vi "scottSSObs.vi"(7 "Observer Variables":T1, 10 "u":dbl, 11 "y":dbl) -> (0 "xhat":dbl[](array[numeric]), 3 "-Kx":dbl)   [LabVIEW 2018, in "kevLib2010.lvlib"]
uses:
  kevLib2010.lvlib
  <vilib>/Analysis/baseanly.llb/Real Dot Product.vi
  <vilib>/Analysis/baseanly.llb/A x Vector.vi
  <vilib>/Analysis/NI_AALBase.lvlib
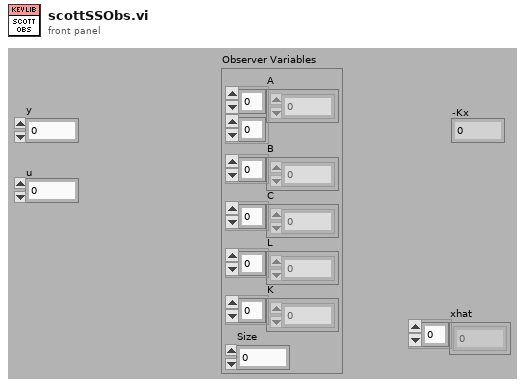
[diagram p1: front panel]
types:
  T1 = cluster{"A":dbl[][], "B":dbl[], "C":dbl[], "L":dbl[], "K":dbl[], "Size":dbl}
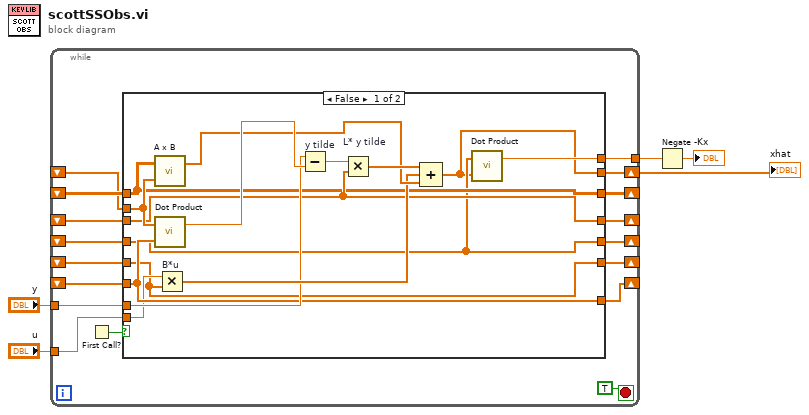
[diagram p0: block diagram]
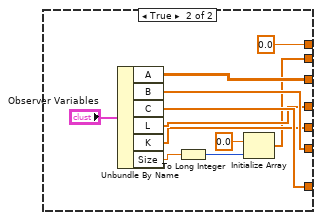
[diagram p2: hidden frame]
diagram:
  n1 = while {
    shift-right: [w20] -> _
    shift-left: _ -> [w15]
    shift-right: [w19] -> _
    shift-left: _ -> [w14]
    shift-right: [w18] -> _
    shift-left: _ -> [w13]
    shift-right: [w17] -> _
    shift-left: _ -> [w12]
    shift-right: [w16] -> _
    shift-left: _ -> [w11]
    shift-right: [w10] -> w1
    shift-left: _ -> [w9]
    tunnel: "y" -> [w8]
    tunnel: "u" -> [w7]
    tunnel: [w6] -> w3
    stop <- TRUE stop-if-true
    n2 = First Call?() -> (First Call?: T/F=w21:bool)
    n3 = case shown="False" w21 {
      tunnel: [w28 w47] -> w20
      tunnel: [w26 w46] -> w19
      tunnel: [w29 w45] -> w18
      tunnel: [w30 w44] -> w17
      tunnel: [w25 w43] -> w16
      tunnel: w15 -> [w28 _]
      tunnel: w14 -> [w26 _]
      tunnel: w13 -> [w29 _]
      tunnel: w12 -> [w30 _]
      tunnel: w11 -> [w25 _]
      tunnel: [w23 w39] -> w10
      tunnel: w9 -> [w31 _]
      tunnel: w8 -> [w32 _]
      tunnel: w7 -> [w27 _]
      tunnel: [w24 0.0 ("X * Y")] -> w6
      frame False {
        n4 = call-poly <vilib>:"A x B.vi"("Vector"=w31, "A"=w28) -> ("A x Vector"=w35:dbl[])  [unwired: 1 out]
        n5 = call-poly <vilib>:"Dot Product.vi"("Y Vector"=w29, "X Vector"=w31) -> ("X * Y"=w37:dbl)  [unwired: 1 out]
        n6 = Multiply "B*u"(x=w27, y=w26) -> (x*y=w34:dbl[])
        n7 = Subtract "y tilde"(x=w32, y=w37) -> (x-y=w33:dbl)
        n8 = Multiply "L* y tilde"(x=w33, y=w30) -> (x*y=w36:dbl[])
        n9 = Compound Arithmetic op=ADD(w36, w34, w35) -> (w23:dbl[])
        n10 = call-poly <vilib>:"Dot Product.vi"("Y Vector"=w23, "X Vector"=w25) -> ("X * Y"=w24:dbl)  [unwired: 1 out]
      }
      frame True {
        n11 = Unbundle By Name("Observer Variables") -> ("A"=w47:dbl[][], "B"=w46:dbl[], "C"=w45:dbl[], "L"=w44:dbl[], "K"=w43:dbl[], "Size"=w41:dbl)
        n12 = To Long Integer(number=w41) -> (32bit integer=w42:i32)
        n13 = Initialize Array(0.0 ("element"), w42) -> (w39:dbl[])
      }
    }
  }
  "xhat" <- w1
  n14 = Negate(x=w3) -> (-x=→"-Kx":dbl)
